vi "Write Config.vi"(8 "error in (no error)":errorcluster, 9 "Re-Init?":bool, 10 "ICM File In":path, 11 "Multiple Queries in":refnum<class "Multiple Queries.lvclass">) -> (0 "error out":errorcluster, 3 "Multiple Queries out":refnum<class "Multiple Queries.lvclass">)   [LabVIEW 2015, in "Multiple Queries.lvclass"]
doc: "Multiple QuerIes.lvclass:Write Config.vi\n\nThis VI writes the Multple Queries Class parameters to the ICM configuration file.\n\nInstrument Communication Module Version 1.0\nDecember, 2017 Original Code Consulting David Thomson\n www.originalcode.com"
uses:
  Multiple Queries.lvclass
  Multiple Queries.lvclass/Multiple Queries.ctl
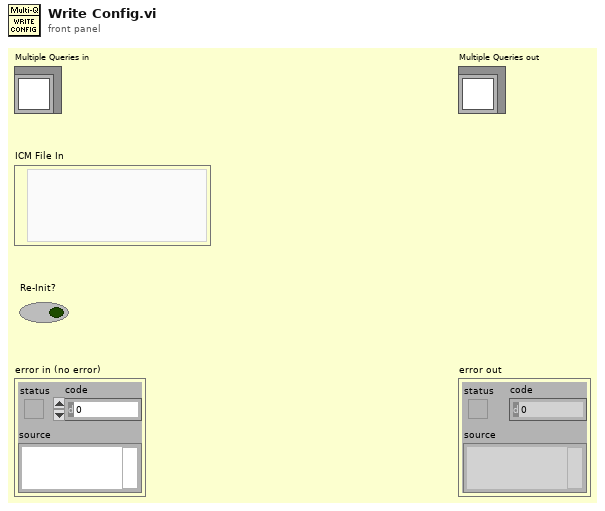
[diagram p1: front panel]
types:
  T1 = typedef "Multiple Queries.lvclass/Multiple Queries Config.ctl" = cluster{"Response Separator":string, "Queries":string[], "Time Between Queries (ms)":u32}
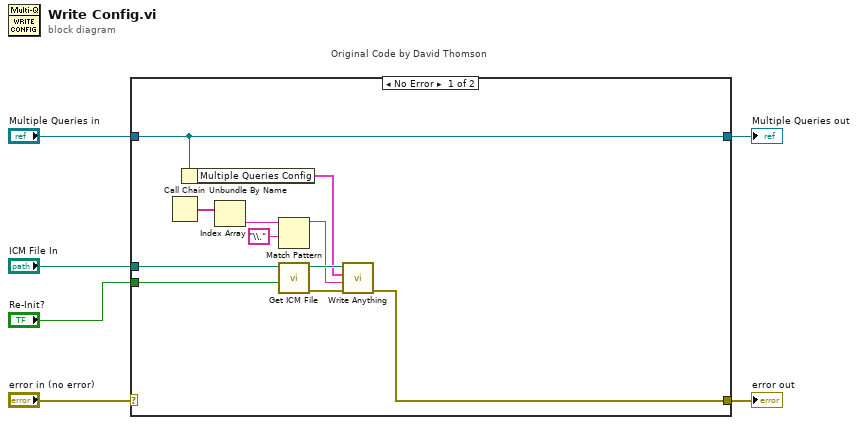
[diagram p0: block diagram]
diagram:
  n1 = case "Original Code by David Thomson" shown="No Error" "error in (no error)" {
    selector: "error in (no error)" -> [_ w19]
    tunnel: [w9 w19] -> w5
    tunnel: [w14 w18] -> w3
    tunnel: "Multiple Queries in" -> [w14 w18]
    tunnel: "ICM File In" -> [w8 _]
    tunnel: "Re-Init?" -> [w7 _]
    frame No Error {
      n2 = Call Chain() -> (call chain=w16:string[])
      n3 = Unbundle By Name(w14) -> ("Multiple Queries Config"=w10:T1)
      n4 = Index Array(array=w16) -> (element=w15:string)  [unwired: 1 in]
      n5 = Match Pattern(string=w15, regular expression="\\.") -> (before substring=w11:string)  [unwired: 1 in, 3 out]
      n6 = call "Get ICM File.vi"("Re-Init?"=w7, "ICM File In"=w8) -> ("error out"=w13:errorcluster, "ICM File"=w12:path)  [unwired: 8 in]
      n7 = call "Write Anything.vi"("Error In"=w13, "Section Name (Name of \"Anything\")"=w11, "Anything"=w10, "Path (dialog)"=w12) -> ("Error Out"=w9:errorcluster)  [unwired: 7 in]
    }
    frame Error {
    }
  }
  "error out" <- w5
  "Multiple Queries out" <- w3
